vi "Autonomous Independent.vi"() -> ()   [LabVIEW 2012]
doc: "This VI is called when autonomous begins, and will automatically be terminated when autonomous ends. You can carry out timed or sensor driven robot movement independently without needing to return to the caller."
uses:
  <vilib>/Rock Robotics/WPI/Relay/WPI_RelayValue.ctl
  <vilib>/Rock Robotics/WPI/RobotDrive/WPI_RobotDriveGetSetRefNum.vi
  Robot Global Data.vi
panel:
  out "Stop Drive":bool
  out "DT Output":enum16{"Off", "Up", "Down"}(ring)=enum."Down"
  out "BAD Up":bool
  out "DAD Output":T1
  out "Shift Low":bool
  out "Feeder Happy":bool
  out "Auton Done":bool
  out "Shooter Happy":bool
  out "Shooter Speed":T2(ring)
  out "Shoot!":bool
  out "Loop Rate (Hz)":dbl
  out "Delay Switch":u32
  out "Seccond Switch":u32
  out "First Switch":u32
  # "Be sure to right-click and choose Data Operations>>Make Current Value default if you want to save the array values with the VI"
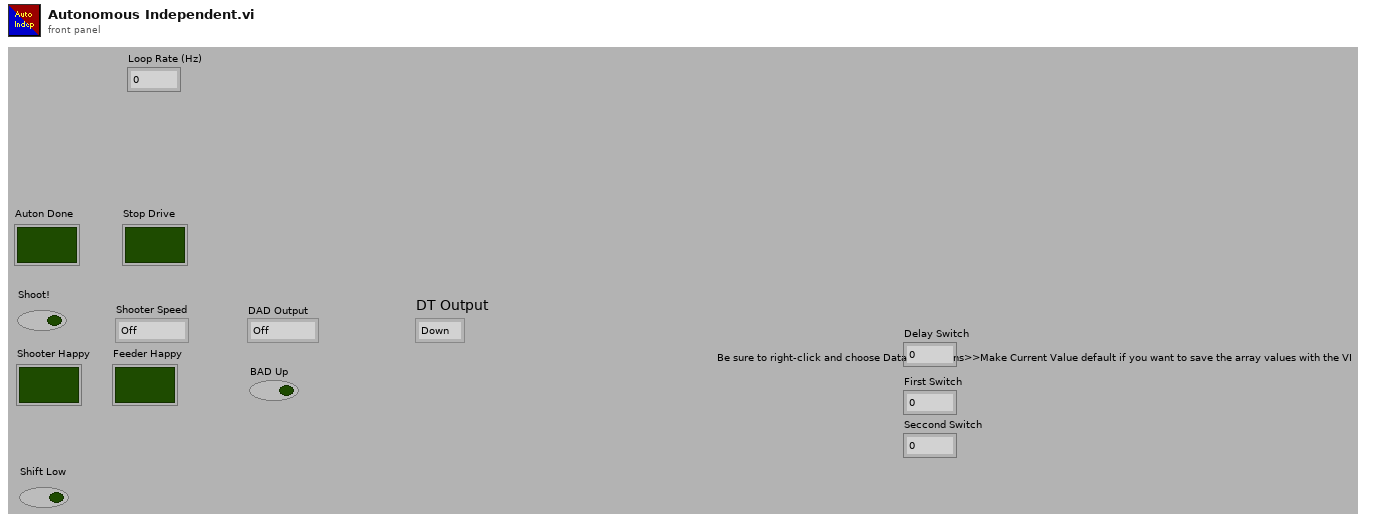
[diagram p1: front panel]
types:
  T1 = typedef "WPI_RelayValue.ctl" = enum16{"Off", "On", "Forward", "Reverse"}
  T2 = enum16{"Off", "2pt Key Shot", "3pt Key Shot", "Back Shot", "Fender Shot", "Key Close", "Key Far"}
  T3 = enum16{"Off", "2pt Key Shot", "3pt Key Shot", "Back Shot", "Fender Shot"}
  T4 = typedef "WPI_RobotDriveDevRef.ctl" = cluster{"DevStatus":errorcluster, "Motors[]":T5[], "Square Inputs":bool, "Max Output":dbl, "Isochronous":bool}
  T5 = typedef "WPI_MotorControlDeviceRef.ctl" = cluster{"DeviceStatus":errorcluster, "Type":enum16{"PWM", "CAN"}, "PWM":cluster{"Digital Module":T6, "PWM Channel":T7, "DeadBand":T8}, "CAN":cluster{"Device Number":u8, "Control Mode":T9, "Semaphore":T10, "Max Vout":dbl}, "Invert":bool, "TransformRef":T11, "InvTransformRef":T11}
  T6 = typedef "FPGA_TypedefDigitalModule.ctl" = enum16{"Digital Module 1", "Digital Module 2"}
  T7 = typedef "FPGA_DIOPWMChannel.ctl" = enum8{"PWM 1", "PWM 2", "PWM 3", "PWM 4", "PWM 5", "PWM 6", "PWM 7", "PWM 8", "PWM 9", "PWM 10", "Invalid"}
  T8 = typedef "WPI_PWMDeadband.ctl" = cluster{"Name":string, "maxPositivePwm":i32, "minPositivePwm":i32, "centerPwm":i32, "maxNegativePwm":i32, "minNegativePwm":i32, "angularRange":u16}
  T9 = typedef "WPI_CANJaguar_ControlMode.ctl" = enum8{"Percent VBus", "Current", "Speed", "Position", "Voltage"}
  T10 = typedef "Semaphore RefNum" = refnum<k1>
  T11 = typedef "WPI_PWMTransform_ConPane.ctl" = refnum<vi>
  T12 = typedef "WPI_GyroDevRef.ctl" = cluster{"DevStatus":errorcluster, "Analog Module":T13, "Analog Channel":T14, "Offset":dbl, "Gain (VoltsPerDegree/Second)":dbl}
  T13 = typedef "FPGA_TypedefAnalogModule.ctl" = enum16{"Analog Module 1", "Analog Module 2"}
  T14 = typedef "FPGA_AIChannel.ctl" = enum8{"AI 1", "AI 2", "AI 3", "AI 4", "AI 5", "AI 6", "AI 7", "AI 8", "Invalid"}
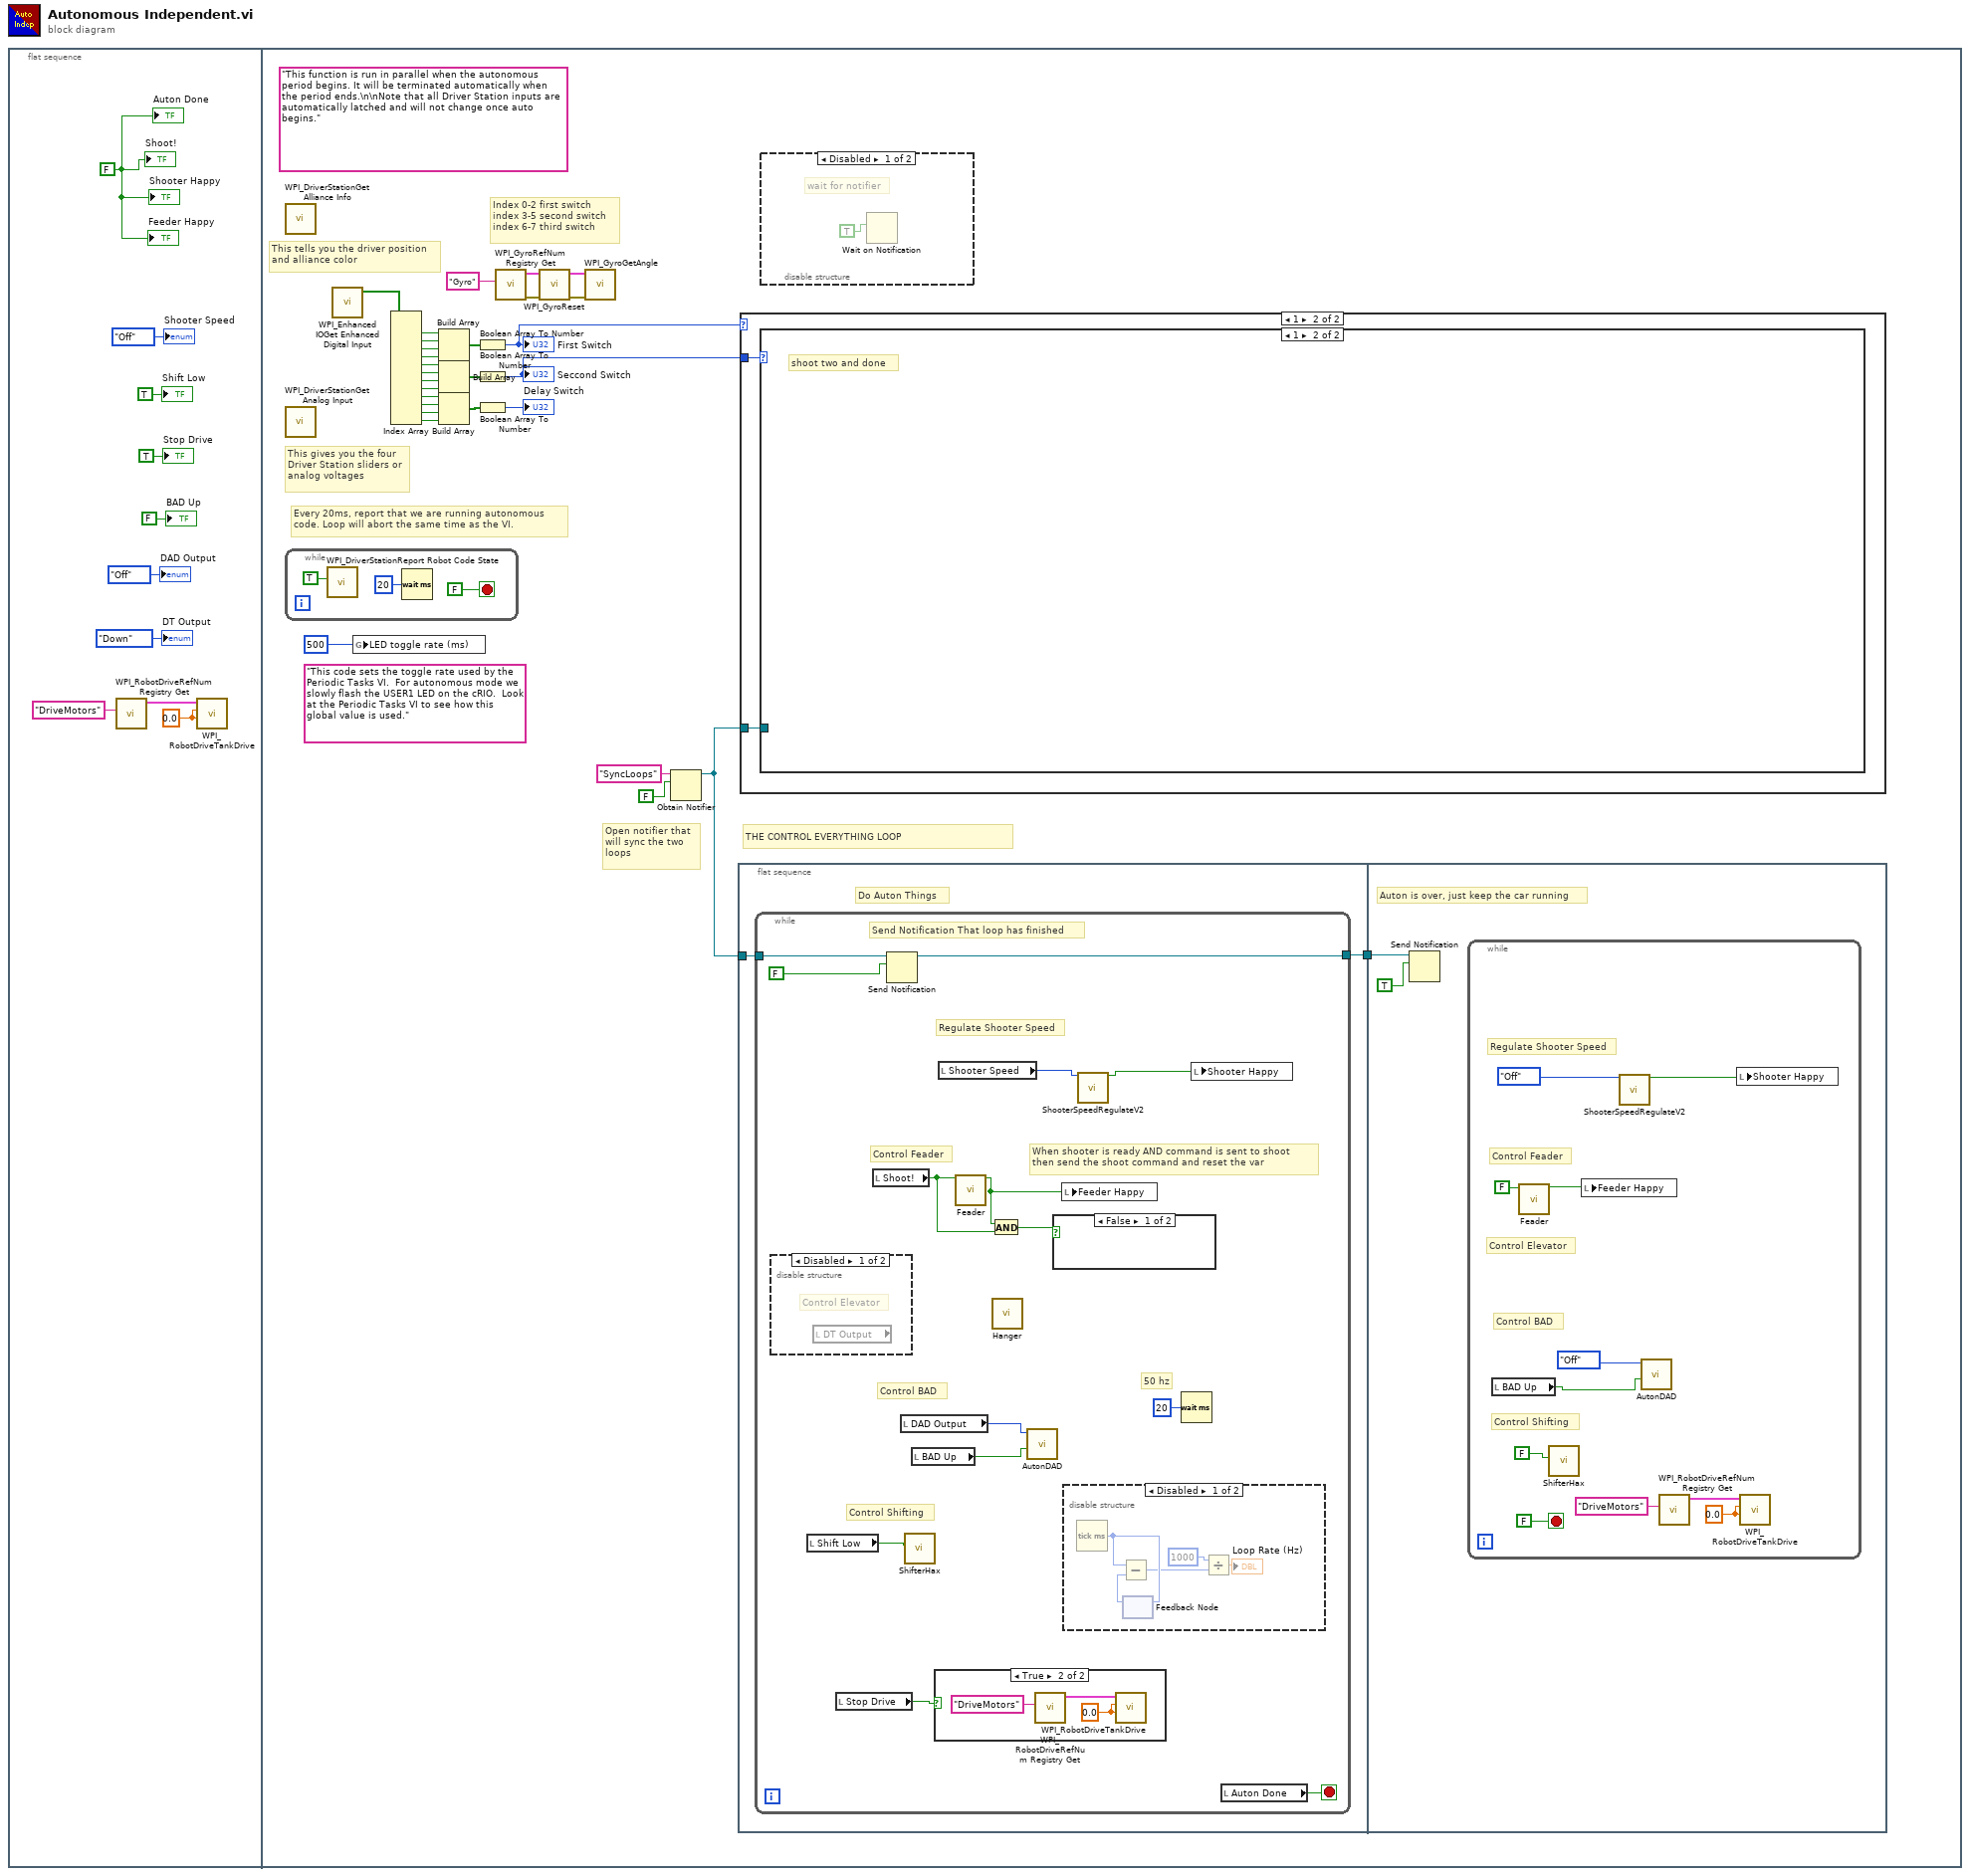
[diagram p0: block diagram]
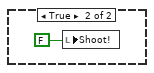
[diagram p6: hidden frame]
diagram:
  n1 = flat-sequence {
    frame #0 {
      w2 = 0.0 ("Left axis value")
      w9 = FALSE
      n2 = call <vilib>:"WPI_RobotDriveRefNum Registry Get.vi"("refnum name"="DriveMotors") -> ("RobotDriveDevRef"=w4:T4)  [unwired: 1 in, 9 out]
      n3 = call <vilib>:"WPI_RobotDriveTankDrive.vi"("Right axis value"=w2, "Left axis value"=w2, "RobotDriveDevRef"=w4) -> ()  [unwired: 6 in, 3 out]
      "Shooter Speed" <- T2."Off" ("Shooter Speed")
      "Feeder Happy" <- w9
      "Shift Low" <- TRUE ("Shift Low")
      "DAD Output" <- WPI_RelayValue."Off" ("DAD Output")
      "BAD Up" <- FALSE ("BAD Up")
      "Stop Drive" <- TRUE ("Stop Drive")
      "Shoot!" <- w9
      "Shooter Happy" <- w9
      "Auton Done" <- w9
      "DT Output" <- enum16{"Off", "Up", "Down"}."Down" ("DT Output")
    }
    frame #1 {
      (unwired) "This code sets the toggle rate used by the Periodic Tasks VI.  For autonomous mode we slowly flash the USER1 LED on the cRIO.  Look at the Periodic Tasks VI to see how this global value is used."
      (unwired) "This function is run in parallel when the autonomous period begins. It will be terminated automatically when the period ends.\n\nNote that all Driver Station inputs are automatically latched and will not change once auto begins."
      # "THE CONTROL EVERYTHING LOOP"
      # "Index 0-2 first switch\nindex 3-5 second switch\nindex 6-7 third switch"
      # "Open notifier that\nwill sync the two\nloops"
      # "Every 20ms, report that we are running autonomous\ncode. Loop will abort the same time as the VI."
      # "This tells you the driver position\nand alliance color"
      # "This gives you the four\nDriver Station sliders or\nanalog voltages"
      n4 = call <vilib>:"WPI_DriverStationGet Alliance Info.vi"() -> ()  [unwired: 12 out]
      n5 = call <vilib>:"WPI_DriverStationGet Analog Input.vi"() -> ()  [unwired: 12 out]
      n6 = while {
        stop <- FALSE stop-if-true
        n7 = call <vilib>:"WPI_DriverStationReport Robot Code State.vi"("Autonomous"=TRUE) -> ()  [unwired: 10 in, 1 out]
        n8 = Wait (ms)(milliseconds to wait=u32 20) -> ()  [unwired: 1 out]
      }
      n9 = call <vilib>:"WPI_Enhanced IOGet Enhanced Digital Input.vi"() -> ("Digital Input [1-16]"=w14:bool[])  [unwired: 10 in, 1 out]
      n10 = global write "Robot Global Data.vi" "LED toggle rate (ms)"(u32 500 ("LED ms toggle rate")) -> ()
      n11 = Index Array(array=w14) -> (element #1=w35:bool, element #2=w34:bool, element #3=w33:bool, element #4=w21:bool, element #5=w32:bool, element #6=w31:bool, element #7=w23:bool, element #8=w22:bool, element #9=w20:bool, element #10=w19:bool, element #11=w18:bool, element #12=w17:bool)  [unwired: 12 in]
      n12 = Build Array(w35, w34, w33, w21) -> (w29:bool[])
      n13 = Build Array(w32, w31, w23, w22) -> (w30:bool[])
      n14 = Build Array(w20, w19, w18, w17) -> (w16:bool[])
      n15 = Boolean Array To Number(Boolean array=w29) -> (number=w13:u32)
      "First Switch" <- w13
      n16 = Boolean Array To Number(Boolean array=w30) -> (number=w12:u32)
      "Seccond Switch" <- w12
      n17 = Boolean Array To Number(Boolean array=w16) -> (number=→"Delay Switch":u32)
      n18 = call <vilib>:"WPI_GyroRefNum Registry Get.vi"("refnum name"="Gyro") -> ("error out"=w24:errorcluster, "GyroDevRef"=w25:T12)  [unwired: 9 in]
      n19 = call <vilib>:"WPI_GyroReset.vi"("error in (no error)"=w24, "GyroDevRef"=w25) -> ("error out"=w27:errorcluster, "GyroDevRef"=w26:T12)  [unwired: 8 in]
      n20 = call <vilib>:"WPI_GyroGetAngle.vi"("error in (no error)"=w27, "GyroDevRef"=w26) -> ()  [unwired: 6 in, 4 out]
      n21 = Obtain Notifier(name (unnamed)="SyncLoops", notification data type=FALSE) -> (notifier out=w11:refnum<notifier>)  [unwired: 2 in, 2 out]
      n22 = flat-sequence {
        tunnel: w11 -> [w43]
        tunnel: [w42] -> w39
        tunnel: w39 -> [w67]
        frame #0 {
          # "Do Auton Things"
          n23 = while {
            tunnel: w43 -> [w55]
            tunnel: [w51] -> w42
            stop <- w57 stop-if-true
            # "Regulate Shooter Speed"
            # "50 hz"
            # "Control BAD"
            # "Control Shifting"
            # "When shooter is ready AND command is sent to shoot\nthen send the shoot command and reset the var"
            # "Control Feader"
            # "Send Notification That loop has finished"
            n24 = disable-structure shown="Disabled" {
              frame Disabled {
                # "Control Elevator"
                n25 = local read "DT Output"() -> ()  [unwired: 1 out]
              }
              frame Enabled {
              }
            }
            n26 = local read "Shift Low"() -> (w46:bool)
            n27 = local read "Stop Drive"() -> (w49:bool)
            n28 = local read "Shoot!"() -> (w54:bool)
            n29 = Send Notification(notification=FALSE, notifier=w55) -> (notifier out=w51:refnum<notifier>)  [unwired: 1 in, 1 out]
            n30 = local read "DAD Output"() -> (w47:T1)
            n31 = call "ShifterHax.vi"("Shifter Button"=w46) -> ()  [unwired: 11 in]
            n32 = local read "BAD Up"() -> (w48:bool)
            n33 = case shown="True" w49 {
              frame False {
              }
              frame True {
                w60 = 0.0 ("Left axis value")
                n34 = call <vilib>:"WPI_RobotDriveRefNum Registry Get.vi"("refnum name"="DriveMotors") -> ("RobotDriveDevRef"=w58:T4)  [unwired: 1 in, 9 out]
                n35 = call <vilib>:"WPI_RobotDriveTankDrive.vi"("Right axis value"=w60, "Left axis value"=w60, "RobotDriveDevRef"=w58) -> ()  [unwired: 6 in, 3 out]
              }
            }
            n36 = local read "Shooter Speed"() -> (w45:T2)
            n37 = call "Feader.vi"("SHOOT Button"=w54) -> ("Ready To Shoot?"=w52:bool)  [unwired: 10 in]
            n38 = And(x=w52, y=w54) -> (x .and. y?=w53:bool)
            n39 = call "Hanger.vi"() -> ()  [unwired: 11 in, 1 out]
            n40 = call "AutonDAD.vi"("BAD UP"=w48, "BAD Output"=w47) -> ()  [unwired: 10 in]
            n41 = case shown="False" w53 {
              frame False {
              }
              frame True {
                n42 = local write "Shoot!"(FALSE) -> ()
              }
            }
            n43 = local write "Feeder Happy"(w52) -> ()
            n44 = disable-structure shown="Disabled" {
              frame Disabled {
                n45 = Tick Count (ms)() -> (millisecond timer value=w65:u32)
                n46 = feedback #1() -> (w64:u32)  [unwired: 1 in]
                n47 = Subtract(x=w65, y=w64) -> (x-y=w62:u32)
                n48 = feedback-in #1(w65) -> ()
                n49 = Divide(x=1000, y=w62) -> (x/y=→"Loop Rate (Hz)":dbl)
              }
              frame Enabled {
              }
            }
            n50 = call "ShooterSpeedRegulateV2.vi"("Shooter Speed"=w45) -> ("ALL GOOD"=w44:bool)  [unwired: 13 in, 1 out]
            n51 = Wait (ms)(milliseconds to wait=u32 20) -> ()  [unwired: 1 out]
            n52 = local write "Shooter Happy"(w44) -> ()
            n53 = local read "Auton Done"() -> (w57:bool)
          }
        }
        frame #1 {
          # "Auton is over, just keep the car running"
          n54 = Send Notification(notification=TRUE, notifier=w67) -> ()  [unwired: 1 in, 2 out]
          n55 = while {
            stop <- FALSE stop-if-true
            w74 = 0.0 ("Left axis value")
            # "Regulate Shooter Speed"
            # "Control BAD"
            # "Control Shifting"
            # "Control Elevator"
            # "Control Feader"
            n56 = local read "BAD Up"() -> (w70:bool)
            n57 = call "Feader.vi"("SHOOT Button"=FALSE) -> ("Ready To Shoot?"=w78:bool)  [unwired: 10 in]
            n58 = call "ShifterHax.vi"("Shifter Button"=FALSE ("Shifting Button")) -> ()  [unwired: 11 in]
            n59 = local write "Feeder Happy"(w78) -> ()
            n60 = call "ShooterSpeedRegulateV2.vi"("Shooter Speed"=T3."Off") -> ("ALL GOOD"=w73:bool)  [unwired: 13 in, 1 out]
            n61 = call "AutonDAD.vi"("BAD UP"=w70, "BAD Output"=WPI_RelayValue."Off") -> ()  [unwired: 10 in]
            n62 = call <vilib>:"WPI_RobotDriveRefNum Registry Get.vi"("refnum name"="DriveMotors") -> ("RobotDriveDevRef"=w76:T4)  [unwired: 1 in, 9 out]
            n63 = local write "Shooter Happy"(w73) -> ()
            n64 = call <vilib>:"WPI_RobotDriveTankDrive.vi"("Right axis value"=w74, "Left axis value"=w74, "RobotDriveDevRef"=w76) -> ()  [unwired: 6 in, 3 out]
          }
        }
      }
      n65 = case shown="1" w13 {
        tunnel: w12 -> [_ w81]
        tunnel: w11 -> [_ w80]
        frame 0, Default {
          # "do nothing"
        }
        frame 1 {
          n66 = case shown="1" w81 {
            tunnel: w80 -> [_ _]
            frame 0, Default {
              # "do nothing"
            }
            frame 1 {
              # "shoot two and done"
            }
          }
        }
      }
      n67 = disable-structure shown="Disabled" {
        frame Disabled {
          # "wait for notifier"
          n68 = Wait on Notification(ignore previous (F)=TRUE) -> (notifier=w41:refnum<notifier>)  [unwired: 2 in, 4 out]
        }
        frame Enabled {
        }
      }
    }
  }
